vi "continue.vi"(0 "连接ID":refnum<k5>) -> (1 "连接ID":refnum<k5>, 2 "输出状态":string)   [LabVIEW 2017]
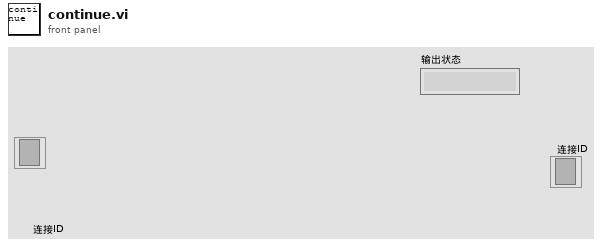
[diagram p1: front panel]
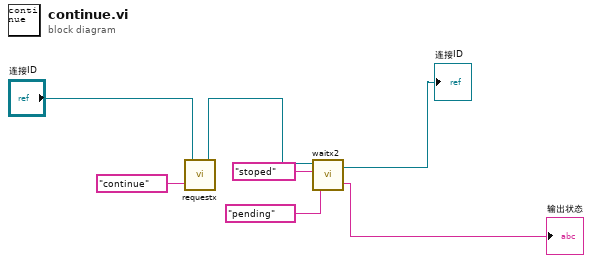
[diagram p0: block diagram]
diagram:
  n1 = call "requestx.vi"("cmd"="continue" ("String"), "连接ID"="连接ID") -> ("连接ID输出"=w5:refnum<k5>)
  n2 = call "waitx2.vi"("String Value 2"="pending", "String Value"="stoped", "连接ID"=w5) -> ("字符串"=→"输出状态":string, "连接ID 2"=→"连接ID":refnum<k5>)  [unwired: 1 in]
